vi "Test Parse Serial Number.vi"(8 "error in (no error)":errorcluster, 11 "Test Case In":refnum<class "Barcode Reader Test.lvclass">) -> (0 "error out":errorcluster, 3 "Test Case Out":refnum<class "Barcode Reader Test.lvclass">)   [LabVIEW 2020, in "Barcode Reader First Iteration.lvlib" / "Barcode Reader Test.lvclass"]
uses:
  Barcode Reader Test.lvclass
  C:/Program Files (x86)/National Instruments/LabVIEW 2020/vi.lib/Astemes/LUnit/Test Case.lvclass
  <vilib>/Astemes/LUnit/Test Case.lvclass/Test Case.ctl
  01074fa8-ee8a-411d-bc8b-fc92c4f90959.vi
  <vilib>/Astemes/LUnit/Palette/Pass.vi
  <vilib>/Astemes/LUnit/Palette/Fail.vi
  <vilib>/Astemes/LUnit/Compare Variants.vi
  <vilib>/Astemes/LUnit/Describe Comparison.vi
  <vilib>/Astemes/LUnit/Set Assertion Type.vi
  <vilib>/Astemes/LUnit/Add test result.vi
  <vilib>/Astemes/LUnit/Variant to string.vi
  <vilib>/Astemes/LUnit/LUnit Record Assertion Result.vi
  <vilib>/Astemes/LUnit/LUnit Aggregate Assertion Results.vi
  <vilib>/Astemes/LUnit/Method Result/LUnit Merge Status.vi
  <vilib>/Astemes/LUnit/LUnit Concatenate result strings.vi
  <vilib>/Utility/Data Type/Get Type Information.vi
  <vilib>/Utility/LVClass/Get LV Class Name.vi
  Barcode Reader/Barcode Reader.lvclass
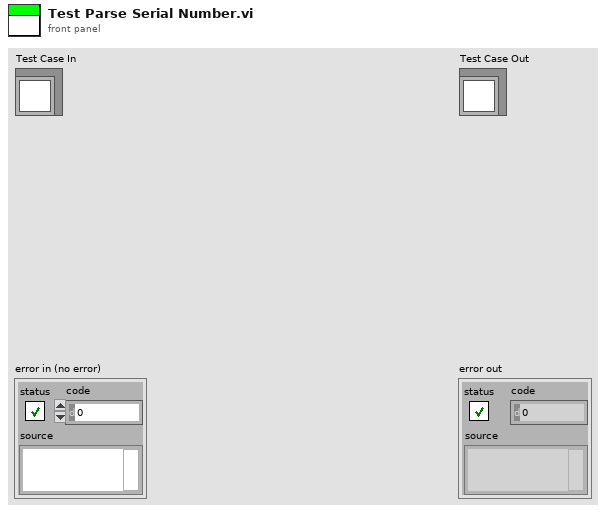
[diagram p1: front panel]
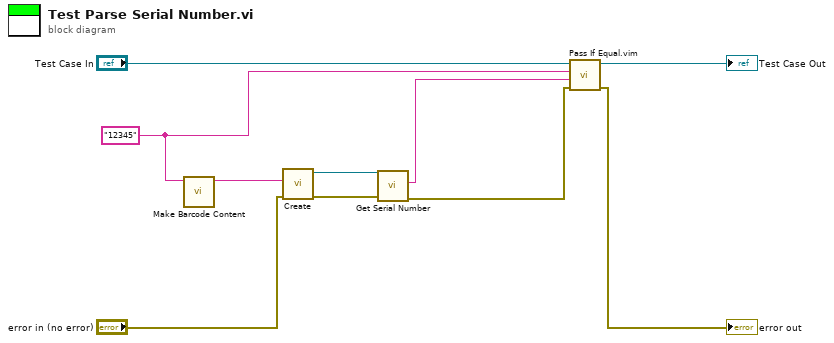
[diagram p0: block diagram]
diagram:
  w1 = "12345" ("Barcode Content")
  n1 = call "Make Barcode Content.vi"("Serial Number"=w1) -> ("Barcode Content"=w7:string)  [unwired: 10 in]
  n2 = call "Create.vi"("error in (no error)"="error in (no error)", "Barcode Content"=w7) -> ("error out"=w4:errorcluster, "Barcode Reader out"=w6:refnum<class "Barcode Reader.lvclass">)  [unwired: 8 in]
  n3 = call "Get Serial Number.vi"("error in (no error)"=w4, "Barcode Reader in"=w6) -> ("error out"=w2:errorcluster, "Serial Number"=w5:string)  [unwired: 7 in, 1 out]
  n4 = call "Pass If Equal.vim"("error in (no error)"=w2, "Actual"=w5, "Expected"=w1, "LUnit Test Case In"="Test Case In") -> ("error out"=→"error out":errorcluster, "LUnit Test Case Out"=→"Test Case Out":refnum<class "Barcode Reader Test.lvclass">)  [unwired: 6 in]
